vi "Set Tuner if Gain.vi"(8 "error in (no error)":errorcluster, 9 "Gain (dB)":dbl, 10 "Stage":i32, 11 "RTL-SDR in":refnum<class "RTL-SDR.lvclass">) -> (0 "error out":errorcluster, 1 "function return":i32, 3 "RTL-SDR out":refnum<class "RTL-SDR.lvclass">)   [LabVIEW 2015, in "RTL-SDR.lvclass"]
uses:
  RTL-SDR.lvclass
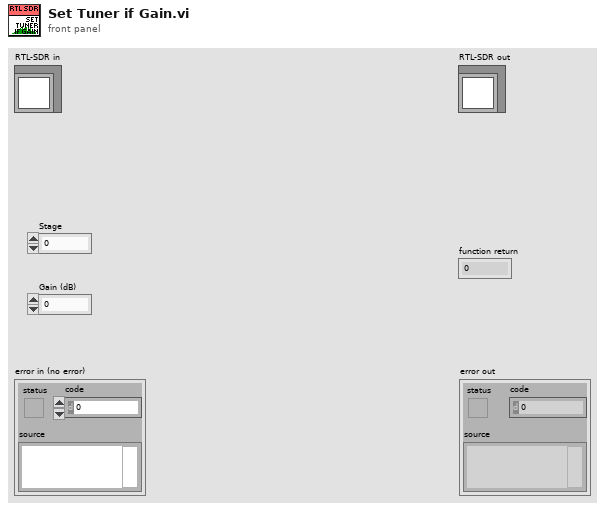
[diagram p1: front panel]
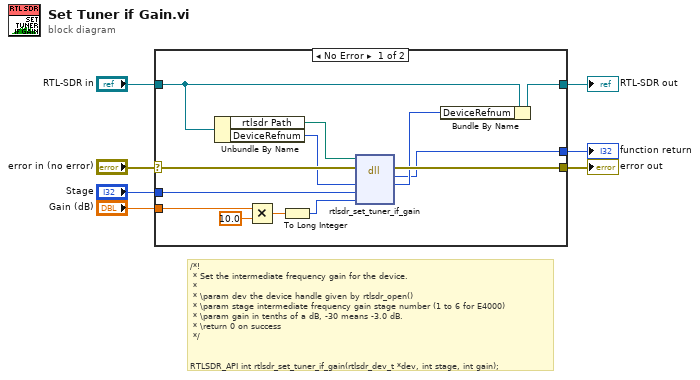
[diagram p0: block diagram]
diagram:
  # "/*!\n * Set the intermediate frequency gain for the device.\n *\n * \\param dev the device handle given by rtlsdr_open()\n * \\param stage intermediate frequency gain stage number (1 to 6 for E4000)\n * \\param gain in tenths of a dB, -30 means -3.0 dB.\n * \\return 0 on success\n */\n\n\nRTLSDR_API int rtlsdr_set_tuner_if_gain(rtlsdr_dev_t *dev, int stage, int gain);"
  n1 = case shown="No Error" "error in (no error)" {
    selector: "error in (no error)" -> [w20 w22]
    tunnel: [w19 w22] -> w6
    tunnel: [w17 w21] -> w4
    tunnel: "RTL-SDR in" -> [w18 w21]
    tunnel: [w13 _] -> w3
    tunnel: "Stage" -> [w12 _]
    tunnel: "Gain (dB)" -> [w8 _]
    frame No Error {
      n2 = Unbundle By Name(w18) -> ("rtlsdr Path"=w16:path, "DeviceRefnum"=w15:u64)
      n3 = Multiply(x=w8, y=10.0) -> (x*y=w11:dbl)
      n4 = To Long Integer(number=w11) -> (32bit integer=w9:i32)
      n5 = dll-call lib="C:/Users/Ivan/Desktop/D-23-09-24 (RTL-SDR)/Project (Pelleng-SDR)/RTL-SDR Class/dll/rtlsdr.*" fn="rtlsdr_set_tuner_if_gain"(path in=w16, error in=w20, "DeviceRefnum"=w15, "Stage"=w12, "Gain"=w9) -> (error out=w19:errorcluster, "return type"=w13:i32, "DeviceRefnum"=w14:u64)  [unwired: 3 in, 1 out]
      n6 = Bundle By Name(cluster=w18, "DeviceRefnum"=w14) -> (w17:refnum<class "RTL-SDR.lvclass">)
    }
    frame Error {
    }
  }
  "error out" <- w6
  "RTL-SDR out" <- w4
  "function return" <- w3
